vi "Log_Append.vi"(2 "Char Size":i32, 5 "To Front(t) End(f)":bool, 7 "Clear":bool, 10 "Sting To Append":string, 11 "String":string) -> (3 "String Out":string)   [LabVIEW 2015]
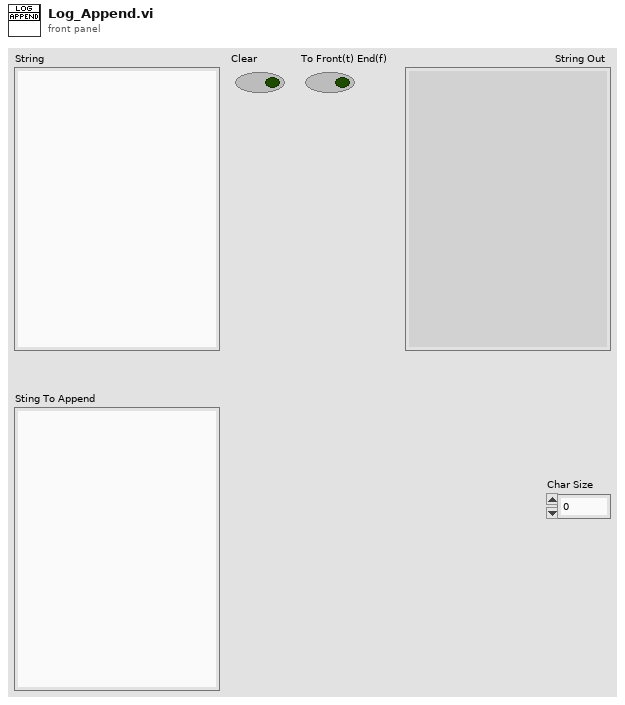
[diagram p1: front panel]
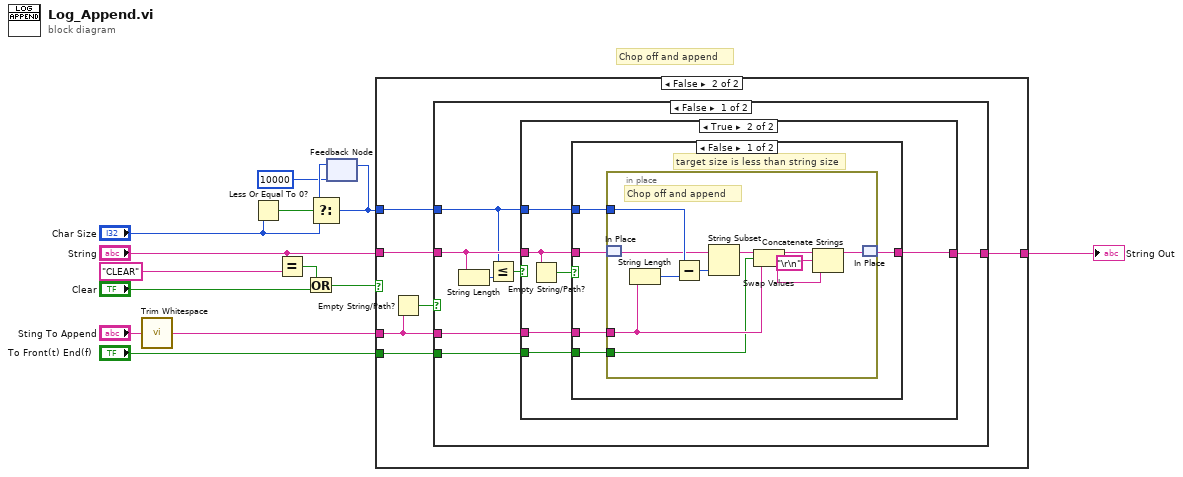
[diagram p0: block diagram]
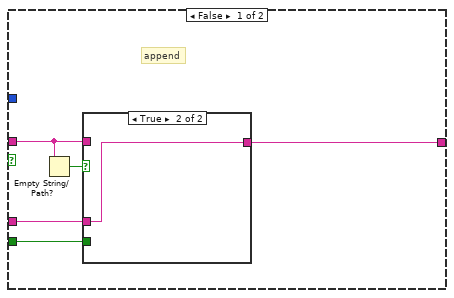
[diagram p3: hidden frame]
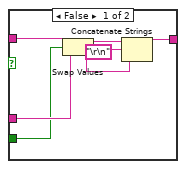
[diagram p4: hidden frame]
diagram:
  # "Chop off and append"
  n1 = call <vilib>:"Trim Whitespace.vi"("string"="Sting To Append") -> ("trimmed string"=w1:string)  [unwired: 1 in]
  n2 = Less Or Equal To 0?(x="Char Size") -> (x <= 0?=w12:bool)
  n3 = Equal?(x="String", y="CLEAR") -> (x = y?=w2:bool)
  n4 = Or(x=w2, y="Clear") -> (x .or. y?=w3:bool)
  n5 = feedback #1(10000 ("Char Size")) -> (w9:i32)
  n6 = Select(t=w9, s=w12, f="Char Size") -> (s? t:f=w10:i32)
  n7 = feedback-in #1(w10) -> ()
  n8 = case shown="False" w3 {
    tunnel: "String" -> [_ w20]
    tunnel: [_ w19] -> w13
    tunnel: w1 -> [_ w16]
    tunnel: w10 -> [_ w18]
    tunnel: "To Front(t) End(f)" -> [_ w17]
    frame True {
      # "CLEAR"
    }
    frame False {
      n9 = Empty String/Path?(string/path=w16) -> (empty?=w15:bool)
      n10 = case shown="False" w15 {
        tunnel: w20 -> [w27 w64]
        tunnel: [w26 w64] -> w19
        tunnel: w18 -> [w24 _]
        tunnel: w17 -> [w22 _]
        tunnel: w16 -> [w21 _]
        frame False {
          n11 = String Length(string=w27) -> (length=w25:i32)
          n12 = Less Or Equal?(x=w24, y=w25) -> (x <= y?=w23:bool)
          n13 = case shown="True" w23 {
            tunnel: w27 -> [w29 w42]
            tunnel: w21 -> [w32 w46]
            tunnel: [w31 w45] -> w26
            tunnel: w24 -> [_ w44]
            tunnel: w22 -> [w30 w43]
            frame False {
              # "append"
              n14 = Empty String/Path?(string/path=w29) -> (empty?=w28:bool)
              n15 = case shown="True" w28 {
                tunnel: w32 -> [w36 w40]
                tunnel: [w35 w40] -> w31
                tunnel: w30 -> [w34 _]
                tunnel: w29 -> [w33 _]
                frame False {
                  n16 = Swap Values(12:w33, 13:w34, 14:w36) -> (1:w38:string, 3:w37:string)
                  n17 = Concatenate Strings(w38, "\r\n", w37) -> (w35:string)
                }
                frame True {
                }
              }
            }
            frame True {
              n18 = Empty String/Path?(string/path=w42) -> (empty?=w41:bool)
              n19 = case shown="False" w41 {
                tunnel: w46 -> [w51 w63]
                tunnel: w42 -> [w50 _]
                tunnel: [w49 w63] -> w45
                tunnel: w44 -> [w48 _]
                tunnel: w43 -> [w47 _]
                frame False {
                  # "target size is less than string size"
                  n20 = in-place {
                    in-place-border: w51 -> [w54]
                    in-place-border: w48 -> [w62]
                    in-place-border: w47 -> [w52]
                    # "Chop off and append"
                    n21 = in-place-match #2(w50) -> (w59:string)
                    n22 = String Length(string=w54) -> (length=w61:i32)
                    n23 = Subtract(x=w62, y=w61) -> (x-y=w60:i32)
                    n24 = String Subset(string=w59, length (rest)=w60) -> (substring=w56:string)  [unwired: 1 in]
                    n25 = Swap Values(12:w56, 13:w52, 14:w54) -> (1:w55:string, 3:w53:string)
                    n26 = Concatenate Strings(w55, "\r\n", w53) -> (w58:string)
                    n27 = in-place-match #2(w58) -> (w49:string)
                  }
                }
                frame True {
                }
              }
            }
          }
        }
        frame True {
        }
      }
    }
  }
  "String Out" <- w13
